vi "SLSC_Command_Out.vi"(6 "SLSC Dynamic Commands":T1[](array[typedef]), 8 "error in":errorcluster, 9 "Values":dbl[](array[numeric]), 10 "session in":refnum<k21>, 11 "SLSC Module Name":refnum<k21>) -> (0 "error out":errorcluster, 2 "session out":refnum<k21>, 3 "SLSC Module Name":refnum<k21>)   [LabVIEW 2015, in "SLSC Module Template Engine.lvlib"]
uses:
  SLSC Module Template Engine.lvlib
  Shared/SLSC Dynamic Channel.ctl
  <vilib>/SLSC/Execute Phys Chan Command.vi
  <vilib>/SLSC/Execute Device Command.vi
  <vilib>/SLSC/SLSC.lvlib
  System Explorer/SLSC Module Template System Explorer.lvlib
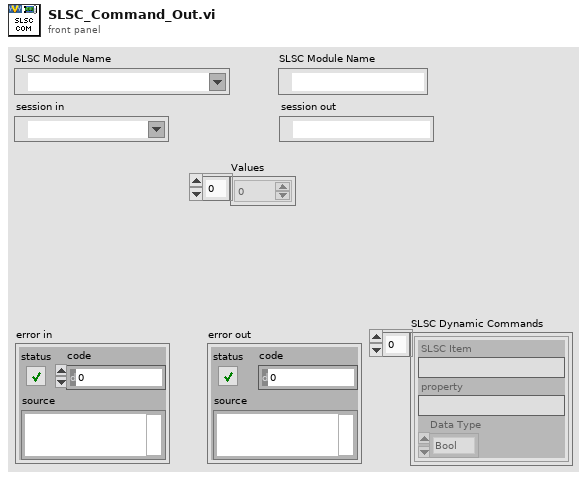
[diagram p1: front panel]
types:
  T1 = typedef "SLSC Module Template System Explorer.lvlib/SLSC Dynamic Channel.ctl" = cluster{"SLSC Item":string, "property":string, "Data Type":enum16{"Bool", "Double", "I32", "I64", "String", "U32", "U64"}}
  T2 = enum16{"Bool", "Double", "I32", "I64", "String", "U32", "U64"}
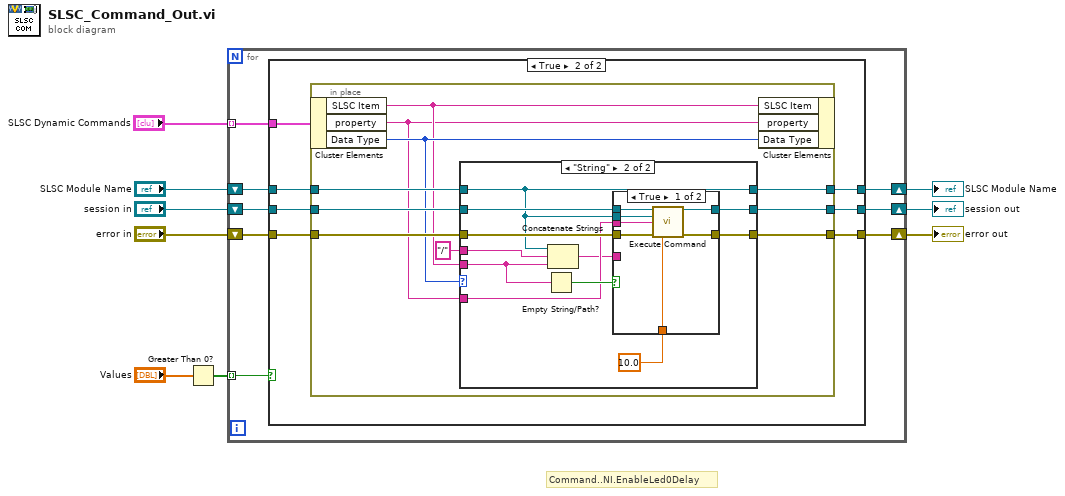
[diagram p0: block diagram]
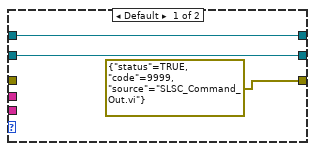
[diagram p3: hidden frame]
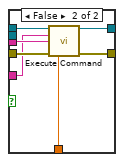
[diagram p4: hidden frame]
diagram:
  # "Command..NI.EnableLed0Delay"
  n1 = Greater Than 0?(x="Values") -> (x > 0?=w1:bool[])
  n2 = for {
    tunnel: "SLSC Dynamic Commands" -> [w17] mode=indexing
    shift-right: [w15] -> w4
    shift-left: "session in" -> [w16]
    shift-right: [w13] -> w6
    shift-left: "SLSC Module Name" -> [w14]
    shift-right: [w11] -> w3
    shift-left: "error in" -> [w12]
    tunnel: w1 -> [w10] mode=indexing
    n3 = case shown="True" w10 {
      tunnel: w17 -> [_ w21]
      tunnel: w16 -> [w19 w27]
      tunnel: [w19 w26] -> w15
      tunnel: w14 -> [w20 w25]
      tunnel: [w20 w24] -> w13
      tunnel: w12 -> [w18 w23]
      tunnel: [w18 w22] -> w11
      frame False {
      }
      frame True {
        n4 = in-place {
          in-place-border: w27 -> [w37]
          in-place-border: [w36] -> w26
          in-place-border: w25 -> [w35]
          in-place-border: [w34] -> w24
          in-place-border: w23 -> [w33]
          in-place-border: [w32] -> w22
          n5 = in-place-cluster #1(w21) -> ("SLSC Item"=w29:string, "property"=w28:string, "Data Type"=w30:T2)
          n6 = case shown="\"String\"" w30 {
            tunnel: w37 -> [w39 w47]
            tunnel: [w39 w50] -> w36
            tunnel: w29 -> [_ w41]
            tunnel: w35 -> [w40 w44]
            tunnel: [w40 w44] -> w34
            tunnel: w33 -> [_ w46]
            tunnel: [errorcluster {"status"=TRUE, "code"=9999, "source"="SLSC_Command_Out.vi"} ("error out") w49] -> w32
            tunnel: "/" -> [_ w51]
            tunnel: w28 -> [_ w43]
            frame Default {
            }
            frame "String" {
              n7 = Empty String/Path?(string/path=w41) -> (empty?=w45:bool)
              n8 = Concatenate Strings(w44, w51, w41) -> (w42:string)
              n9 = case shown="True" w45 {
                tunnel: w47 -> [w58 w65]
                tunnel: [w57 w64] -> w50
                tunnel: [w56 w63] -> w49
                tunnel: 10.0 ("timeout (10 sec)") -> [w55 w62]
                tunnel: w46 -> [w54 w61]
                tunnel: w43 -> [w53 w60]
                tunnel: w42 -> [_ w59]
                tunnel: w44 -> [w52 _]
                frame True {
                  n10 = call-poly <vilib>:"Execute Command.vi"("session in"=w58, "devices"=w52, "command"=w53, "error in (no error)"=w54, "timeout (10 sec)"=w55) -> ("session out"=w57:refnum<k21>, "error out"=w56:errorcluster)  [unwired: 9 in]
                }
                frame False {
                  n11 = call-poly <vilib>:"Execute Command.vi"("session in"=w65, "physical channels"=w59, "command"=w60, "error in (no error)"=w61, "timeout (10 sec)"=w62) -> ("session out"=w64:refnum<k21>, "error out"=w63:errorcluster)  [unwired: 9 in]
                }
              }
            }
          }
          n12 = in-place-cluster #1("SLSC Item"=w29, "property"=w28, "Data Type"=w30) -> ()  [unwired: 1 out]
        }
      }
    }
  }
  "error out" <- w3
  "session out" <- w4
  "SLSC Module Name" <- w6
